vi "Fade_Into_Color.vi"(9 "Color_Goal":u32(colorbox)=16776002, 10 "Color_Start":u32(colorbox)=16776002, 11 "fade constant":dbl) -> ()   [LabVIEW 2020]
uses:
  5d26372a-a2b6-4d3c-a03a-b0bed839a150.vi
  LED/Global-Led.vi
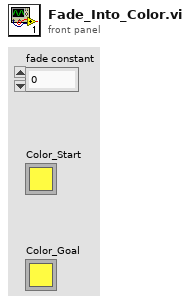
[diagram p1: front panel]
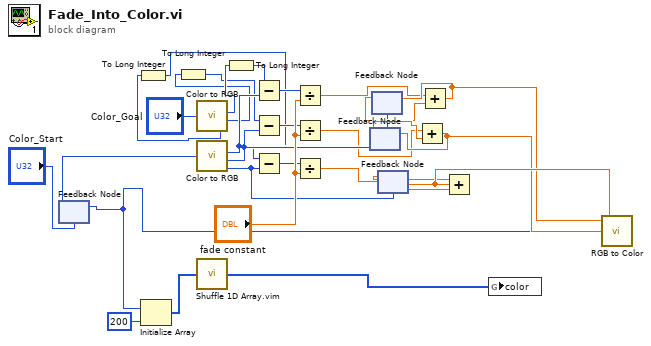
[diagram p0: block diagram]
diagram:
  n1 = feedback #1("Color_Start") -> (w5:u32)
  n2 = call <vilib>:"Color to RGB.vi"("Color"="Color_Goal") -> ("R"=w13:u8, "G"=w11:u8, "B"=w9:u8)  [unwired: 1 out]
  n3 = To Long Integer(number=w9) -> (32bit integer=w8:i32)
  n4 = To Long Integer(number=w11) -> (32bit integer=w10:i32)
  n5 = call <vilib>:"Color to RGB.vi"("Color"=w5) -> ("R"=w20:u8, "G"=w23:u8, "B"=w26:u8)  [unwired: 1 out]
  n6 = To Long Integer(number=w13) -> (32bit integer=w12:i32)
  n7 = Subtract(x=w12, y=w20) -> (x-y=w15:i32)
  n8 = Subtract(x=w10, y=w23) -> (x-y=w16:i32)
  n9 = Subtract(x=w8, y=w26) -> (x-y=w17:i32)
  n10 = Divide(x=w15, y="fade constant") -> (x/y=w4:dbl)
  n11 = Divide(x=w16, y="fade constant") -> (x/y=w3:dbl)
  n12 = Divide(x=w17, y="fade constant") -> (x/y=w2:dbl)
  n13 = feedback #2(w23) -> (w24:dbl)
  n14 = feedback #3(w20) -> (w21:dbl)
  n15 = feedback #4(w26) -> (w27:dbl)
  n16 = Add(x=w3, y=w24) -> (x+y=w25:dbl)
  n17 = feedback-in #2(w25) -> ()
  n18 = Add(x=w4, y=w21) -> (x+y=w22:dbl)
  n19 = feedback-in #3(w22) -> ()
  n20 = Add(x=w27, y=w2) -> (x+y=w28:dbl)
  n21 = feedback-in #4(w28) -> ()
  n22 = call <vilib>:"RGB to Color.vi"("B"=w28, "G"=w25, "R"=w22) -> ("Color"=w6:u32)
  n23 = feedback-in #1(w6) -> ()
  n24 = Initialize Array(w6, 200 ("dimension size")) -> (w19:u32[])
  n25 = call "Shuffle 1D Array.vim"("array"=w19) -> ("shuffled array"=w1:u32[])  [unwired: 4 in]
  n26 = global write "Global-Led.vi" "color"(w1) -> ()
